vi "Bad Cluster elements warning.vi"(8 "error in (no error)":errorcluster, 11 "Error items":string[](array[string])) -> (0 "error out":errorcluster)   [LabVIEW 2020, in "Library Commun.lvlib" / "Variant JSON.lvlib"]
uses:
  Variant JSON.lvlib
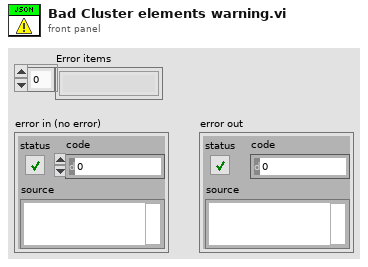
[diagram p1: front panel]
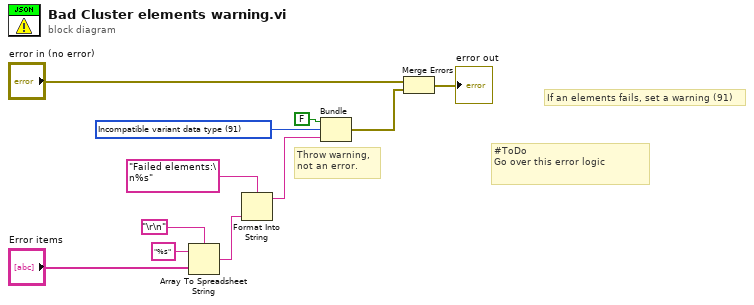
[diagram p0: block diagram]
diagram:
  w7 = 91 items=["No error", "Argument error", "Memory is full", "Out of zone", "End of file", "File already open", "Generic file I/O error", "File not found", "File permission error", "Disk is full", "Duplicate path", "Too many files open", "System feature not enabled", "Resource file not found", "Cannot add resource", "Resource not found", "Image not found", "Image memory error", "Pen does not exist", "Config type invalid", "Config token not found", "Config parse error", "Config memory error", "Bad external code format", "Bad external code offset", "External code not present", "Null window", "Destroy window error", "Null menu", "Print aborted", "Bad print record", "Print driver error", "Windows error during printing", "Memory error during printing", "Print dialog error", "Generic print error", "Invalid device refnum", "Device not found", "Device parameter error", "Device unit error", "Cannot open device", "Device call aborted", "Generic error", "Cancelled by user", "Object ID too low", "Object ID too high", "Object not in heap", "Unknown heap", "Unknown object (invalid DefProc)", "Unknown object (DefProc not in table)", "Message out of range", "Invalid (null) method", "Unknown message", "Manager call not supported", "Bad address", "Network operation in progress", "Network operation timed out", "Connection is busy", "Network attribute not supported", "Network error", "Address in use", "System out of memory", "Connection aborted", "Connection refused", "Not connected", "Already connected", "Connection closed", "Initialization error (interapplication manager)", "Bad occurrence", "Wait on unbound occurrence handler", "Occurrence queue overflow", "Datalog type conflict", "Unused", "Unrecognized type (interapplication manager)", "Memory corrupt", "Failed to make temporary DLL", "Old CIN version", "Drag socket not found", "Failed to load drop-object", "Failed to register OLE object", "Failed to release OLE object", "Format specifier type mismatch", "Unknown format specifier", "Too few format specifiers", "Too many format specifiers", "Scan failed", "Newer CIN version", "Error converting to variant", "Runtime menu error", "Password tampered", "Variant attribute not found", "Incompatible variant data type", "Event data is not available", "Event Store is not present", "Occurrence is not found", "Event Queue is not created", "Event info is not available", "Refnum passed is NULL", "Error retrieving Class GUID", "Error retrieving CoClass GUID", "Error retrieving TypeLib GUID.", "Bad built application magic bytes.", "Specific driver is different from the specific driver associated with the Logical Name.", "There is no session opened to the class driver.", "Max Error", "MAX - Error with config objects", "MAX - Error loading configuration", "MAX - Group not supported"]
  # "If an elements fails, set a warning (91)"
  # "#ToDo\nGo over this error logic"
  # "Throw warning,\nnot an error."
  n1 = Array To Spreadsheet String(delimiter (Tab)="\r\n", array="Error items", 3:"%s" ("format string")) -> (spreadsheet string=w4:string)
  n2 = Format Into String(format string="Failed elements:\n%s", w4) -> (resulting string=w5:string)  [unwired: 2 in, 1 out]
  n3 = Bundle("empty?"=FALSE, w7, w5) -> (w10:cluster{"empty?":bool, i32, string})  [unwired: 1 in]
  n4 = Merge Errors("error in (no error)", w10) -> (→"error out":errorcluster)
